vi "Call Vector Field Histogram.vi"(0 "LIDAR magn. (m)":dbl[](array[numeric]), 1 "max speed":dbl=0.7, 2 "Initialize?":bool, 5 "LIDAR angle (rad)":dbl[](array[numeric]), 7 "current heading (deg)":dbl, 9 "target heading (deg)":dbl, 11 "target distance":dbl, 12 "obstacle clearance (m)":dbl, 13 "thresholds":T1) -> (4 "command vx":dbl, 6 "command vy":dbl, 8 "command heading (deg)":dbl, 10 "histogram out":dbl[](array[numeric]), 15 "mask out":bool[](array[boolean]))   [LabVIEW 2012]
uses:
  <vilib>/Analysis/coordinate.llb/Angle Rotation (scalar).vi
  <vilib>/Analysis/coordinate.llb/Wrap Angle (scalar).vi
  <vilib>/Utility/AngleManip/Degrees to Radians (Scalar DBL).vi
  <vilib>/Utility/AngleManip/Radians to Degrees (Scalar DBL).vi
  <vilib>/robotics/Obstacle Avoidance/Advanced Vector Field Histogram/NI_Robotics_Vector Field Histogram.lvlib
  <vilib>/Utility/AngleManip/NI_AngleManipulation.lvlib
  <vilib>/Analysis/NI_AAL_Angle.lvlib
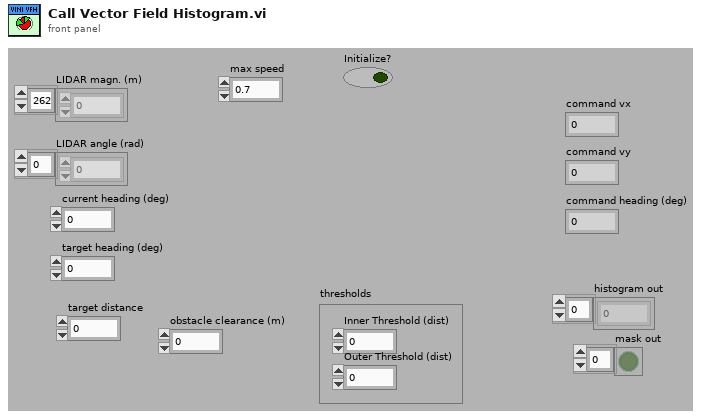
[diagram p1: front panel]
types:
  T1 = cluster{"Inner Threshold (dist)":dbl, "Outer Threshold (dist) ":dbl}
  T2 = cluster{"current heading (deg)":dbl, "target heading (deg)":dbl}
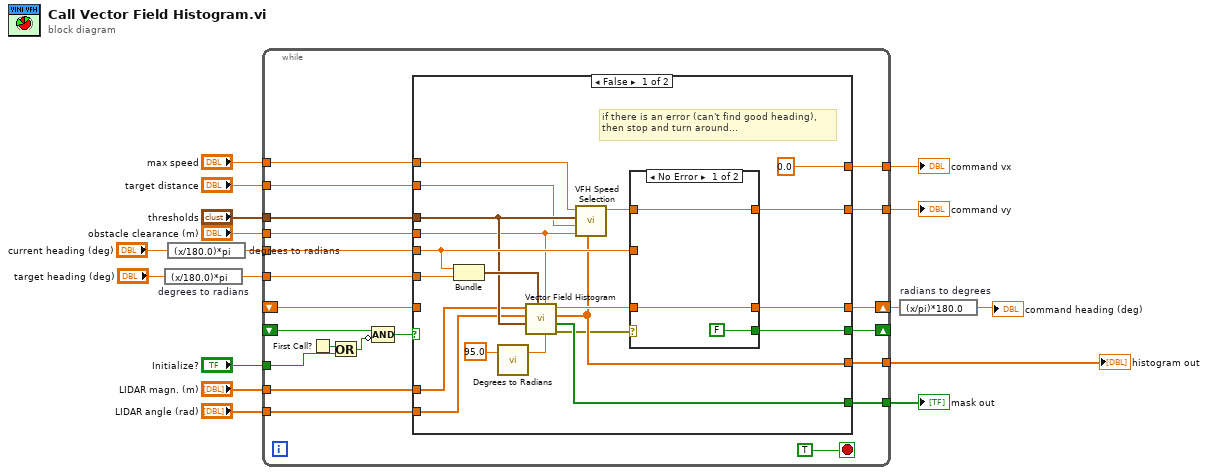
[diagram p0: block diagram]
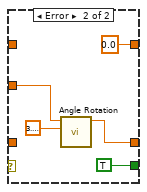
[diagram p2: hidden frame]
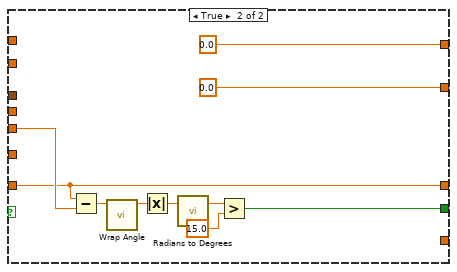
[diagram p3: hidden frame]
diagram:
  n1 = expression code="(x/180.0)*pi" "degrees to radians"("target heading (deg)") -> (w2:dbl)
  n2 = expression code="(x/180.0)*pi" "degrees to radians"("current heading (deg)") -> (w3:dbl)
  n3 = while {
    tunnel: [w37] -> w16
    tunnel: "max speed" -> [w36]
    tunnel: [w35] -> w14
    tunnel: w3 -> [w34]
    tunnel: [w33] -> w12
    shift-right: [w30] -> _
    shift-left: _ -> [w26]
    shift-right: [w29] -> w11
    shift-left: _ -> [w28]
    tunnel: [w38] -> w17
    tunnel: "thresholds" -> [w24]
    tunnel: "target distance" -> [w23]
    tunnel: "obstacle clearance (m)" -> [w22]
    tunnel: w2 -> [w21]
    tunnel: "LIDAR angle (rad)" -> [w20]
    tunnel: "LIDAR magn. (m)" -> [w19]
    tunnel: "Initialize?" -> [w18]
    stop <- TRUE stop-if-true
    n4 = First Call?() -> (First Call?: T/F=w31:bool)
    n5 = Or(x=w31, y=w18) -> (x .or. y?=w27:bool)
    n6 = Compound Arithmetic op=AND(w26, invert w27) -> (w25:bool)
    n7 = case shown="False" w25 {
      tunnel: [w58 0.0 ("VX")] -> w38
      tunnel: [0.0 0.0] -> w37
      tunnel: w36 -> [w55 _]
      tunnel: [w50 _] -> w35
      tunnel: w34 -> [w51 w74]
      tunnel: [w56 _] -> w33
      tunnel: [w49 w72] -> w30
      tunnel: [w53 w71] -> w29
      tunnel: w28 -> [_ w71]
      tunnel: w24 -> [w44 _]
      tunnel: w23 -> [w43 _]
      tunnel: w22 -> [w42 _]
      tunnel: w21 -> [w41 _]
      tunnel: w20 -> [w40 _]
      tunnel: w19 -> [w39 _]
      frame False {
        # "if there is an error (can't find good heading),\nthen stop and turn around..."
        n8 = Bundle("current heading (deg)"=w51, "target heading (deg)"=w41) -> (w47:T2)  [unwired: 1 in]
        n9 = call-poly <vilib>:"Degrees to Radians.vi"("angle (deg)"=95.0) -> ("angle (rad)"=w45:dbl)  [unwired: 2 in]
        n10 = call <vilib>:"Vector Field Histogram.vi"("maximum heading change (rad)"=w45, "obstacle clearance distance"=w42, "heading"=w47, "thresholds"=w44, "direction angles (rad)"=w40, "distances"=w39) -> ("error out"=w48:errorcluster, "mask"=w56:bool[], "histogram"=w50:dbl[], "chosen heading (rad)"=w54:dbl)  [unwired: 2 in]
        n11 = call "VFH Speed Selection.vi"("Histogram"=w50, "Obstacle Clearance"=w42, "Target Distance"=w43, "Thresholds"=w44, "Max Speed"=w55) -> ("Speed"=w52:dbl)  [unwired: 6 in]
        n12 = case shown="No Error" w48 {
          tunnel: [w60 0.0 ("VX")] -> w58
          tunnel: w54 -> [w61 _]
          tunnel: [w61 w62] -> w53
          tunnel: w52 -> [w60 _]
          tunnel: w51 -> [_ w64]
          tunnel: [FALSE TRUE] -> w49
          frame No Error {
          }
          frame Error {
            n13 = call-poly <vilib>:"Angle Rotation.vi"("counterclockwise rotation"=3.141592653589793, "angle"=w64) -> ("rotated angle"=w62:dbl)  [unwired: 8 in, 1 out]
          }
        }
      }
      frame True {
        n14 = Subtract(x=w71, y=w74) -> (x-y=w68:dbl)
        n15 = call-poly <vilib>:"Wrap Angle.vi"("angle in"=w68) -> ("angle out"=w67:dbl)  [unwired: 9 in, 1 out]
        n16 = Absolute Value(x=w67) -> (abs(x)=w70:dbl)
        n17 = call-poly <vilib>:"Radians to Degrees.vi"("angle (rad)"=w70) -> ("angle (deg)"=w69:dbl)  [unwired: 2 in]
        n18 = Greater?(x=w69, y=15.0) -> (0:w72:bool)
      }
    }
  }
  "command vy" <- w17
  "command vx" <- w16
  "histogram out" <- w14
  "mask out" <- w12
  n19 = expression code="(x/pi)*180.0" "radians to degrees"(w11) -> (→"command heading (deg)":dbl)
